vi "Begin.vi"(11 "Image Size":T1=enum."160x120") -> (0 "error out":errorcluster)   [LabVIEW 2013]
doc: "Called before other user functions, this VI is expected to open initial I/O refnums, load in file data, and do all program initialization. Notice that the <B>error out</B> terminal is simply used for data flow. Wiring it to other structures or subVIs ensures that this VI runs first."
uses:
  <vilib>/Rock Robotics/WPI/Camera/WPI_CameraImageSize.ctl
  <vilib>/Rock Robotics/SystemInterfaces/DIO/FPGA_DIOPWMChannel.ctl
  <vilib>/Rock Robotics/WPI/SafetyOutput/WPI_SafetyOutputConfigMenu.ctl
  <vilib>/Rock Robotics/WPI/DriverStation/WPI_DriverStationRobotMode2.ctl
  <vilib>/Rock Robotics/WPI/Joystick/WPI_JoystickDeviceEnum.ctl
  <vilib>/Rock Robotics/SystemInterfaces/DIO/FPGA_DIOChannel.ctl
  <vilib>/Rock Robotics/SystemInterfaces/DIO/FPGA_DIORelayChannel.ctl
  <vilib>/Rock Robotics/WPI/Solenoid/WPI_SolenoidChannel.ctl
  <vilib>/Rock Robotics/WPI/RobotDrive/WPI_RobotDriveOpen2MotorWithTalon.vi
  Robot Global Data.vi
  <vilib>/Rock Robotics/WPI/MotorControl/WPI_MotorControlOpen Talon.vi
  <vilib>/Rock Robotics/WPI/Solenoid/WPI_SolenoidOpenSingle.vi
  <vilib>/Rock Robotics/WPI/Compressor/WPI_CompressorGetSetRefNum.vi
  <vilib>/Rock Robotics/WPI/Camera/WPI_CameraWhite Balance Values.ctl
  <vilib>/Rock Robotics/WPI/Camera/WPI_CameraExposure Values.ctl
  <vilib>/Rock Robotics/WPI/Camera/WPI_CameraFrameRate.ctl
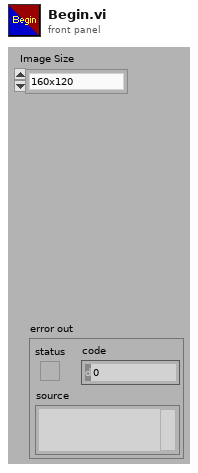
[diagram p1: front panel]
types:
  T1 = typedef "WPI_CameraImageSize.ctl" = enum16{"640x480", "320x240", "160x120"}
  T2 = typedef "WPI_SolenoidChannel.ctl" = enum8{"Solenoid 1", "Solenoid 2", "Solenoid 3", "Solenoid 4", "Solenoid 5", "Solenoid 6", "Solenoid 7", "Solenoid 8", "Invalid"}
  T3 = typedef "FPGA_DIOChannel.ctl" = enum8{"DIO 1", "DIO 2", "DIO 3", "DIO 4", "DIO 5", "DIO 6", "DIO 7", "DIO 8", "DIO 9", "DIO 10", "DIO 11", "DIO 12", "DIO 13", "DIO 14", "Invalid"}
  T4 = typedef "FPGA_DIORelayChannel.ctl" = enum8{"Relay 1", "Relay 2", "Relay 3", "Relay 4", "Relay 5", "Relay 6", "Relay 7", "Relay 8", "Invalid"}
  T5 = typedef "WPI_JoystickDeviceEnum.ctl" = enum16{"USB 1", "USB 2", "USB 3", "USB 4", "Kinect 1", "Kinect 2"}
  T6 = typedef "FPGA_DIOPWMChannel.ctl" = enum8{"PWM 1", "PWM 2", "PWM 3", "PWM 4", "PWM 5", "PWM 6", "PWM 7", "PWM 8", "PWM 9", "PWM 10", "Invalid"}
  T7 = typedef "WPI_DriverStationRobotMode2.ctl" = enum16{"Autonomous Disabled", "Autonomous Enabled", "Teleop Disabled", "Teleop Enabled", "Timeout", "Finish", "Test Disabled", "Test Enabled"}
  T8 = typedef "WPI_SafetyOutputConfigMenu.ctl" = enum16{"Enable", "Disable"}
  T9 = typedef "WPI_CameraFrameRate.ctl" = u32
  T10 = typedef "WPI_CameraExposure Values.ctl" = enum16{"Auto", "Flicker-free 50 Hz", "Flicker-free 60 Hz", "Hold current"}
  T11 = typedef "WPI_CameraWhite Balance Values.ctl" = enum16{"Auto", "Fixed indoor", "Fixed outdoor 1", "Fixed outdoor 2", "Fixed fluorescent 1", "Fixed fluorescent 2", "Hold current"}
  T12 = typedef "WPI_CameraDevRef.ctl" = cluster{"Camera Address":string, "CameraStatus":errorcluster, "Acquire Image Notifier":refnum<notifier>}
  T13 = typedef "WPI_MotorControlDeviceRef.ctl" = cluster{"DeviceStatus":errorcluster, "Type":enum16{"PWM", "CAN"}, "PWM":cluster{"Digital Module":T14, "PWM Channel":T6, "DeadBand":T15}, "CAN":cluster{"Device Number":u8, "Control Mode":T16, "Semaphore":T17, "Max Vout":dbl}, "Invert":bool, "TransformRef":T18, "InvTransformRef":T18}
  T14 = typedef "FPGA_TypedefDigitalModule.ctl" = enum16{"Digital Module 1", "Digital Module 2"}
  T15 = typedef "WPI_PWMDeadband.ctl" = cluster{"Name":string, "maxPositivePwm":i32, "minPositivePwm":i32, "centerPwm":i32, "maxNegativePwm":i32, "minNegativePwm":i32, "angularRange":u16}
  T16 = typedef "WPI_CANJaguar_ControlMode.ctl" = enum8{"Percent VBus", "Current", "Speed", "Position", "Voltage"}
  T17 = typedef "Semaphore RefNum" = refnum<k1>
  T18 = typedef "WPI_PWMTransform_ConPane.ctl" = refnum<vi>
  T19 = typedef "WPI_DigitalInputDevRef.ctl" = cluster{"DevStatus":errorcluster, "DIO Channel":T3, "Digital Module":T14}
  T20 = typedef "WPI_SolenoidDevRef.ctl" = cluster{"DevStatus":errorcluster, "Solenoid Module":T21, "Forward Solenoid Channel":T2, "Reverse Solenoid Channel":T2}
  T21 = typedef "FPGA_TypedefSolenoidModule.ctl" = enum16{"Solenoid Module 1", "Solenoid Module 2"}
  T22 = typedef "WPI_CompressorDevRef.ctl" = cluster{"DevStatus":errorcluster, "DigitalInputDevRef":T19, "RelayDevRef":T23}
  T23 = typedef "WPI_RelayDevRef.ctl" = cluster{"DevStatus":errorcluster, "Relay Channel":T4, "Digital Module":T14, "Relay Direction":T24}
  T24 = typedef "WPI_RelayDirection.ctl" = enum16{"Both directions", "Forward only", "Reverse only"}
  T25 = typedef "WPI_JoystickDevRef.ctl" = cluster{"Device":T5}
  T26 = typedef "WPI_RobotDriveDevRef.ctl" = cluster{"DevStatus":errorcluster, "Motors[]":T13[], "Square Inputs":bool, "Max Output":dbl, "Isochronous":bool}
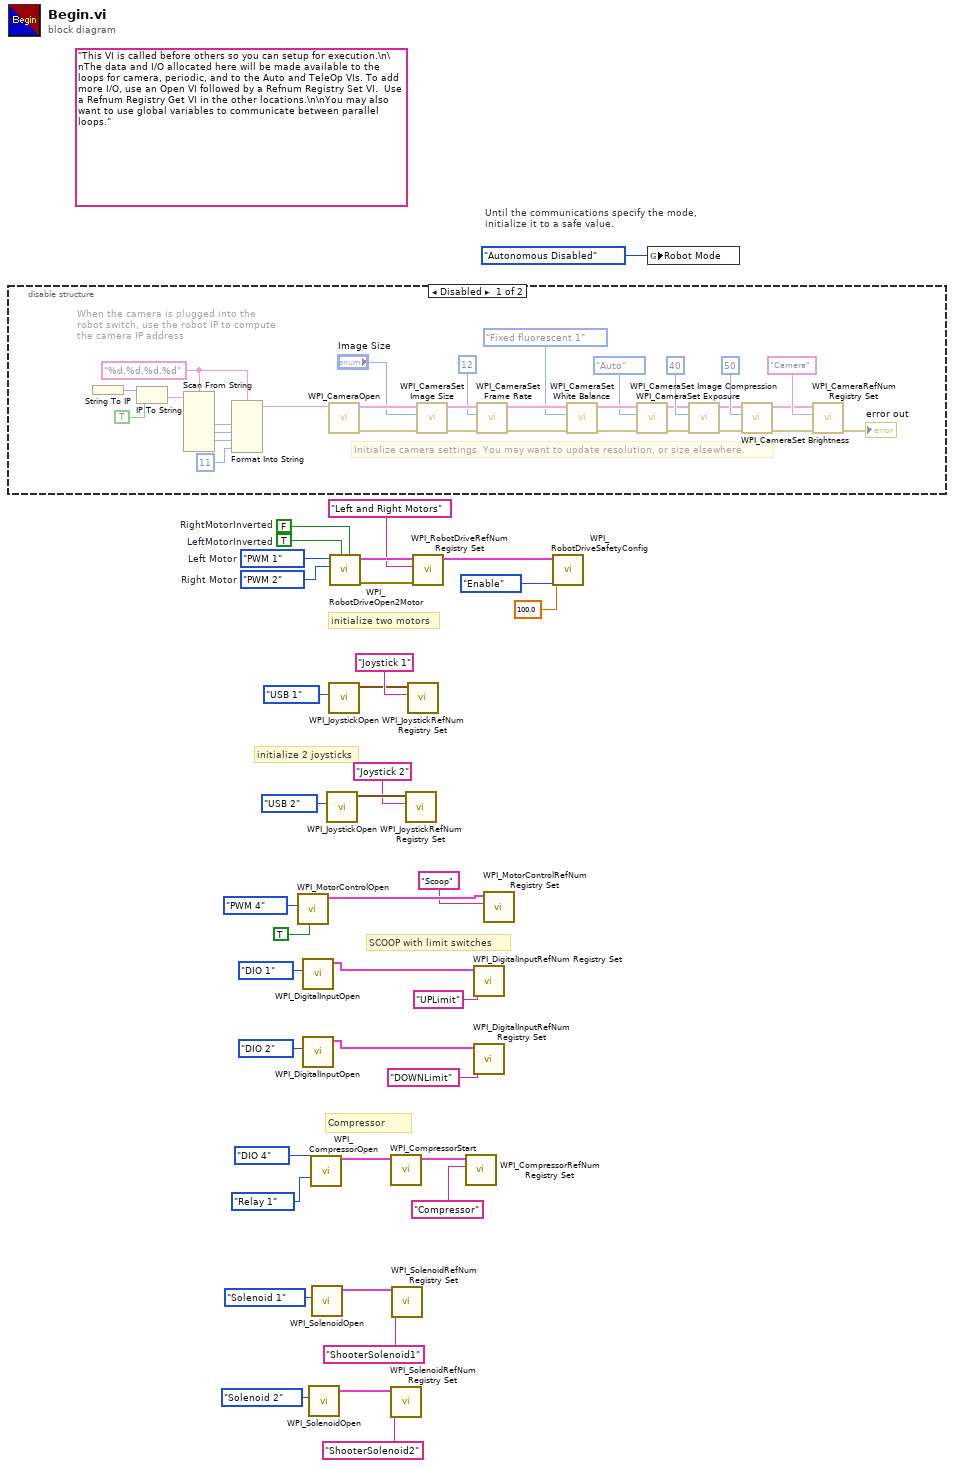
[diagram p0: block diagram]
diagram:
  (unwired) "This VI is called before others so you can setup for execution.\n\nThe data and I/O allocated here will be made available to the loops for camera, periodic, and to the Auto and TeleOp VIs. To add more I/O, use an Open VI followed by a Refnum Registry Set VI.  Use a Refnum Registry Get VI in the other locations.\n\nYou may also want to use global variables to communicate between parallel loops."
  w32 = FPGA_DIOPWMChannel."PWM 2"  # Right Motor
  w33 = FPGA_DIOPWMChannel."PWM 1"  # Left Motor
  w37 = TRUE  # LeftMotorInverted
  w38 = FALSE  # RightMotorInverted
  # "SCOOP with limit switches"
  # "Compressor"
  # "initialize 2 joysticks"
  # "Until the communications specify the mode,\ninitialize it to a safe value."
  # "initialize two motors"
  n1 = disable-structure shown="Disabled" {
    frame Disabled {
      w41 = "%d.%d.%d.%d" ("format string")
      # "When the camera is plugged into the\nrobot switch, use the robot IP to compute\nthe camera IP address"
      # "Initialize camera settings. You may want to update resolution, or size elsewhere."
      n2 = String To IP() -> (0:w48:u32)  [unwired: 1 in]
      n3 = IP To String(1:TRUE ("dot notation? (F)"), 2:w48) -> (0:w46:string)
      n4 = Scan From String(format string=w41, input string=w46) -> (output 1=w45:i32, output 2=w44:i32, output 3=w43:i32)  [unwired: 7 in, 3 out]
      n5 = Format Into String(format string=w41, w45, w44, w43, 11 ("Compression")) -> (resulting string=w40:string)  [unwired: 2 in, 1 out]
      n6 = call <vilib>:"WPI_CameraOpen.vi"("Camera Address"=w40) -> ("error out"=w60:errorcluster, "CameraDevRef"=w61:T12)  [unwired: 1 in, 8 out]
      n7 = call <vilib>:"WPI_CameraSet Image Size.vi"("error in (no error)"=w60, "Image Size"="Image Size", "CameraDevRef"=w61) -> ("error out"=w59:errorcluster, "CameraDevRef Out"=w62:T12)  [unwired: 7 out]
      n8 = call <vilib>:"WPI_CameraSet Frame Rate.vi"("error in (no error)"=w59, "Frame Rate (fps)"=T9 12, "CameraDevRef"=w62) -> ("error out"=w58:errorcluster, "CameraDevRef Out"=w64:T12)  [unwired: 7 out]
      n9 = call <vilib>:"WPI_CameraSet White Balance.vi"("error in (no error)"=w58, "White Balance"=WPI_CameraWhite_Balance_Values."Fixed fluorescent 1", "CameraDevRef"=w64) -> ("error out"=w57:errorcluster, "CameraDevRef Out"=w63:T12)  [unwired: 7 out]
      n10 = call <vilib>:"WPI_CameraSet Exposure.vi"("error in (no error)"=w57, "Exposure"=WPI_CameraExposure_Values."Auto", "CameraDevRef"=w63) -> ("error out"=w56:errorcluster, "CameraDevRef Out"=w66:T12)  [unwired: 7 out]
      n11 = call <vilib>:"WPI_CameraSet Image Compression.vi"("error in (no error)"=w56, "Compression"=40, "CameraDevRef"=w66) -> ("error out"=w55:errorcluster, "CameraDevRef Out"=w65:T12)  [unwired: 7 out]
      n12 = call <vilib>:"WPI_CameraSet Brightness.vi"("error in (no error)"=w55, "Brightness"=50, "CameraDevRef"=w65) -> ("error out"=w53:errorcluster, "CameraDevRef Out"=w54:T12)  [unwired: 7 out]
      n13 = call <vilib>:"WPI_CameraRefNum Registry Set.vi"("error in (no error)"=w53, "refnum name"="Camera", "CameraDevRef"=w54) -> ("error out"=→"error out":errorcluster)  [unwired: 8 out]
    }
    frame Enabled {
    }
  }
  n14 = call-poly <vilib>:"WPI_MotorControlOpen.vi"("Invert"=TRUE, "PWM Channel"=FPGA_DIOPWMChannel."PWM 4") -> ("MotorControlDeviceRef"=w24:T13)  [unwired: 8 in, 1 out]
  n15 = call <vilib>:"WPI_DigitalInputOpen.vi"("DIO Channel"=FPGA_DIOChannel."DIO 1") -> ("DigitalInputDevRef"=w22:T19)  [unwired: 9 in, 1 out]
  n16 = call <vilib>:"WPI_DigitalInputOpen.vi"("DIO Channel"=FPGA_DIOChannel."DIO 2") -> ("DigitalInputDevRef"=w17:T19)  [unwired: 9 in, 1 out]
  n17 = call-poly <vilib>:"WPI_SolenoidOpen.vi"("Solenoid Channel"=WPI_SolenoidChannel."Solenoid 2") -> ("SolenoidDevRef"=w4:T20)  [unwired: 9 in, 1 out]
  n18 = call <vilib>:"WPI_CompressorOpen.vi"("Pressure Switch DIO Channel"=FPGA_DIOChannel."DIO 4", "Relay Channel"=FPGA_DIORelayChannel."Relay 1") -> ("CompressorDevRef"=w9:T22)  [unwired: 12 in, 1 out]
  n19 = call-poly <vilib>:"WPI_SolenoidOpen.vi"("Solenoid Channel"=WPI_SolenoidChannel."Solenoid 1") -> ("SolenoidDevRef"=w7:T20)  [unwired: 9 in, 1 out]
  n20 = call <vilib>:"WPI_JoystickOpen.vi"("JoystickDevice"=WPI_JoystickDeviceEnum."USB 2") -> ("JoystickDevRef"=w14:T25)  [unwired: 10 in]
  n21 = call <vilib>:"WPI_JoystickOpen.vi"("JoystickDevice"=WPI_JoystickDeviceEnum."USB 1") -> ("JoystickDevRef"=w27:T25)  [unwired: 10 in]
  n22 = call-poly <vilib>:"WPI_RobotDriveOpen2Motor.vi"("Right Motor Inverted"=w38, "Left Motor Inverted"=w37, "Right Motor"=w32, "Left Motor"=w33) -> ("error out"=w34:errorcluster, "RobotDriveDevRef"=w36:T26)  [unwired: 1 in, 5 out]
  n23 = call <vilib>:"WPI_CompressorStart.vi"("CompressorDevRef"=w9) -> ("CompressorDevRef"=w8:T22)  [unwired: 9 in, 1 out]
  n24 = call <vilib>:"WPI_SolenoidRefNum Registry Set.vi"("refnum name"="ShooterSolenoid2", "SolenoidDevRef"=w4) -> ()  [unwired: 8 in, 2 out]
  n25 = call <vilib>:"WPI_SolenoidRefNum Registry Set.vi"("refnum name"="ShooterSolenoid1", "SolenoidDevRef"=w7) -> ()  [unwired: 8 in, 2 out]
  n26 = call <vilib>:"WPI_JoystickRefNum Registry Set.vi"("refnum name"="Joystick 2", "JoystickDevRef"=w14) -> ()  [unwired: 8 in, 2 out]
  n27 = call <vilib>:"WPI_JoystickRefNum Registry Set.vi"("refnum name"="Joystick 1", "JoystickDevRef"=w27) -> ()  [unwired: 8 in, 2 out]
  n28 = call <vilib>:"WPI_RobotDriveRefNum Registry Set.vi"("error in (no error)"=w34, "refnum name"="Left and Right Motors", "RobotDriveDevRef"=w36) -> ("RobotDriveDevRef"=w31:T26)  [unwired: 8 out]
  n29 = call <vilib>:"WPI_CompressorRefNum Registry Set.vi"("refnum name"="Compressor", "CompressorDevRef"=w8) -> ()  [unwired: 8 in, 2 out]
  n30 = call <vilib>:"WPI_DigitalInputRefNum Registry Set.vi"("refnum name"="UPLimit", "DigitalInputDevRef"=w22) -> ()  [unwired: 8 in, 2 out]
  n31 = call <vilib>:"WPI_DigitalInputRefNum Registry Set.vi"("refnum name"="DOWNLimit", "DigitalInputDevRef"=w17) -> ()  [unwired: 8 in, 2 out]
  n32 = call <vilib>:"WPI_MotorControlRefNum Registry Set.vi"("refnum name"="Scoop", "MotorControlDevRef"=w24) -> ()  [unwired: 8 in, 2 out]
  n33 = call <vilib>:"WPI_RobotDriveSafetyConfig.vi"("timeout (s)"=100.0, "mode"=WPI_SafetyOutputConfigMenu."Enable", "RobotDriveDevRef"=w31) -> ()  [unwired: 7 in, 2 out]
  n34 = global write "Robot Global Data.vi" "Robot Mode"(WPI_DriverStationRobotMode2."Autonomous Disabled" ("Robot Mode")) -> ()
